vi "Home.vi"(8 "error in (no error)":errorcluster, 10 "shutdown":refnum<user-event>, 11 "Modules":T3) -> (0 "error out":errorcluster)   [LabVIEW 2025]
uses:
  Controls/refresh button 2.ctl
  Controls/Test list.ctl
  <vilib>/Handler Framework/CmdQueue/Enqueue Single.vi
  <vilib>/Handler Framework/Handler Framework.lvlib
  Libraries/Motor/Motor.lvlib
panel:
  out "error out 2":errorcluster
  in  "Test Selection":T1
  in  "Refresh":T2
  in  "Program":u16(ring) items=["Start", "Angle", "Return to Home", "End"]
  # "Home"
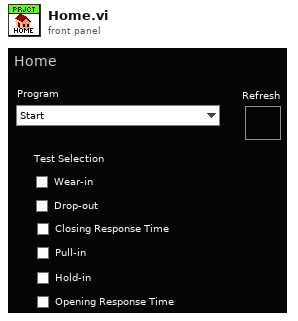
[diagram p1: front panel]
types:
  T1 = typedef "Test list.ctl" = cluster{"Wear-in":bool, "Drop-out":bool, "Closing Response Time":bool, "Pull-in":bool, "Hold-in":bool, "Opening Response Time":bool}
  T2 = typedef "refresh button 2.ctl" = bool
  T3 = cluster{"Module IDs":i32[], "Module Names":string[]}
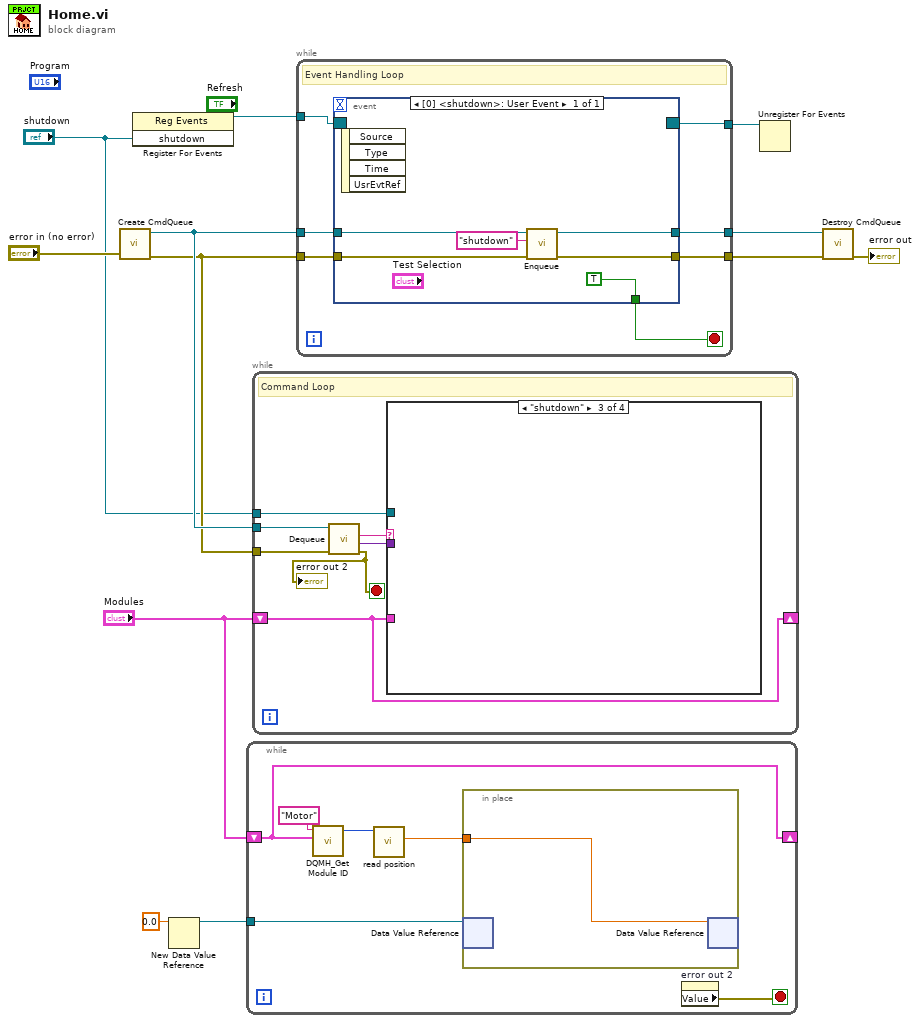
[diagram p0: block diagram]
diagram:
  n1 = call <vilib>:"Create CmdQueue.vi"("error in (no error)"="error in (no error)") -> ("error out"=w9:errorcluster, "CmdQueue out"=w10:refnum<queue>)  [unwired: 9 in]
  n2 = register-events("shutdown") -> (reference out=w8:refnum<event-registration>)  [unwired: 2 in, 1 out]
  n3 = New Data Value Reference(data value=0.0) -> (data value reference=w1:refnum<data-value>)  [unwired: 1 in, 1 out]
  n4 = while {
    shift-right: [w14] -> _
    shift-left: "Modules" -> [w14]
    tunnel: w1 -> [w16]
    stop <- w13 stop-if-true
    n5 = call "DQMH_Get Module ID.vi"("Modules"=w14, "Module Name"="Motor") -> ("Module ID out"=w17:i32)  [unwired: 9 in]
    n6 = call "read position.vi"("Module ID"=w17) -> ("Position"=w15:dbl)  [unwired: 8 in, 2 out]
    n7 = in-place {
      in-place-border: w15 -> [w19]
      n8 = in-place-dvr #1(w16) -> ()  [unwired: 2 out]
      n9 = in-place-dvr #1(w19) -> ()  [unwired: 2 out]
    }
    n10 = property on="error out 2" class="Clust (strict)"() -> ("Value"=w13:errorcluster)  [unwired: 2 in, 2 out]
  }
  n11 = while {
    tunnel: w10 -> [w26]
    tunnel: w9 -> [w22]
    tunnel: "shutdown" -> [w21]
    shift-right: [w20] -> _
    shift-left: "Modules" -> [w20]
    stop <- w23 stop-if-true
    # "Command Loop"
    n12 = call <vilib>:"Dequeue.vi"("error in (no error)"=w22, "CmdQueue in"=w26) -> ("error out"=w23:errorcluster, "value"=w24:variant, "cmd"=w25:string)  [unwired: 5 in, 2 out]
    "error out 2" <- w23
    n13 = case shown="\"shutdown\"" w25 {
      tunnel: w24 -> [_ _ _ _]
      tunnel: w21 -> [_ _ _ _]
      tunnel: w20 -> [_ _ _ _]
      frame "False", Default {
      }
      frame "init" {
      }
      frame "shutdown" {
      }
      frame "refresh" {
      }
    }
  }
  n14 = while {
    tunnel: w10 -> [w33]
    tunnel: [w32] -> w12
    tunnel: w9 -> [w31]
    tunnel: [w30] -> w11
    tunnel: w8 -> [w28]
    tunnel: [w27] -> w7
    stop <- w29 stop-if-true
    # "Event Handling Loop"
    n15 = event shown="[0] <shutdown>: User Event" {
      selector: w28 -> [_]
      dyn-events: [_] -> w27
      timeout: _ -> [_]
      tunnel: w33 -> [w39]
      tunnel: [w38] -> w32
      tunnel: w31 -> [w37]
      tunnel: [w36] -> w30
      tunnel: [TRUE ("Discard?")] -> w29
      event User Event {
        n16 = event-data() -> ()  [unwired: 1 in, 4 out]
        n17 = call-poly <vilib>:"Enqueue.vi"("error in (no error)"=w37, "Command"="shutdown", "CmdQueue in"=w39) -> ("error out"=w36:errorcluster, "CmdQueue out"=w38:refnum<queue>)  [unwired: 7 in]
      }
    }
  }
  n18 = Unregister For Events(event registration refnum=w7) -> ()  [unwired: 1 in, 1 out]
  n19 = call <vilib>:"Destroy CmdQueue.vi"("error in (no error)"=w11, "CmdQueue in"=w12) -> ("error out"=→"error out":errorcluster)  [unwired: 9 in]
